vi "hold_data.vi"(7 "holda_data_mod":T2, 8 "Error In":errorcluster, 10 "config":T1={"rate"=1652.0, "duration"=1.0, "thr"=100.0, "preTrigger"=100.0, "cutoff"=-3.0, "Filtro"=enum."Desativado", "highPass"=1000.0, "lowPass"=1000.0, "updateTime"=50.0} {"updateTime" format="%#_g ms"; "lowPass" format="%#_g Hz"; "highPass" format="%#_g Hz"; "cutoff" format="%#_g dB"; "preTrigger" format="%#_g ms"; "thr" format="%#_g N"; "duration" format="%#_g s"; "rate" min=1652.0 max=51200.0 format="%#_g Hz"}, 11 "data":dbl[][](array[numeric])) -> (0 "Error Out":errorcluster, 3 "finished":bool)   [LabVIEW 2016]
uses:
  hold_data_mods.ctl
  MainFGV/Settings/Advanced/AdvancedConfig.ctl
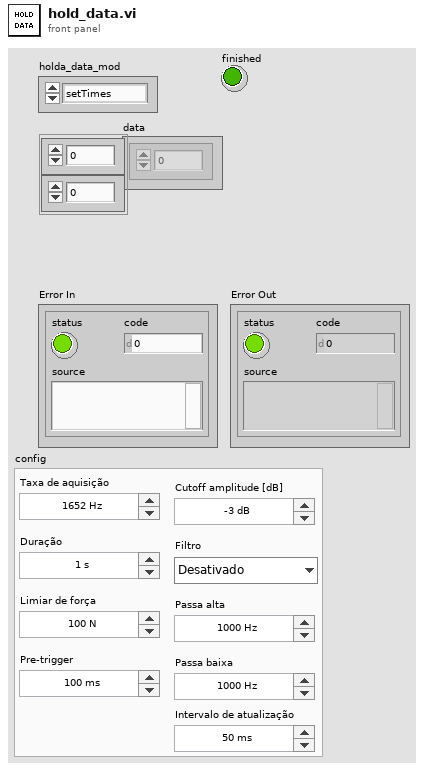
[diagram p1: front panel]
types:
  T1 = typedef "AdvancedConfig.ctl" = cluster{"rate":dbl, "duration":dbl, "thr":dbl, "preTrigger":dbl, "cutoff":dbl, "Filtro":enum16{"Desativado", "Passa banda", "Passa alta", "Passa baixa"}, "highPass":dbl, "lowPass":dbl, "updateTime":dbl}
  T2 = typedef "hold_data_mods.ctl" = enum16{"setTimes", "HoldPreTrigger", "HoldData"}
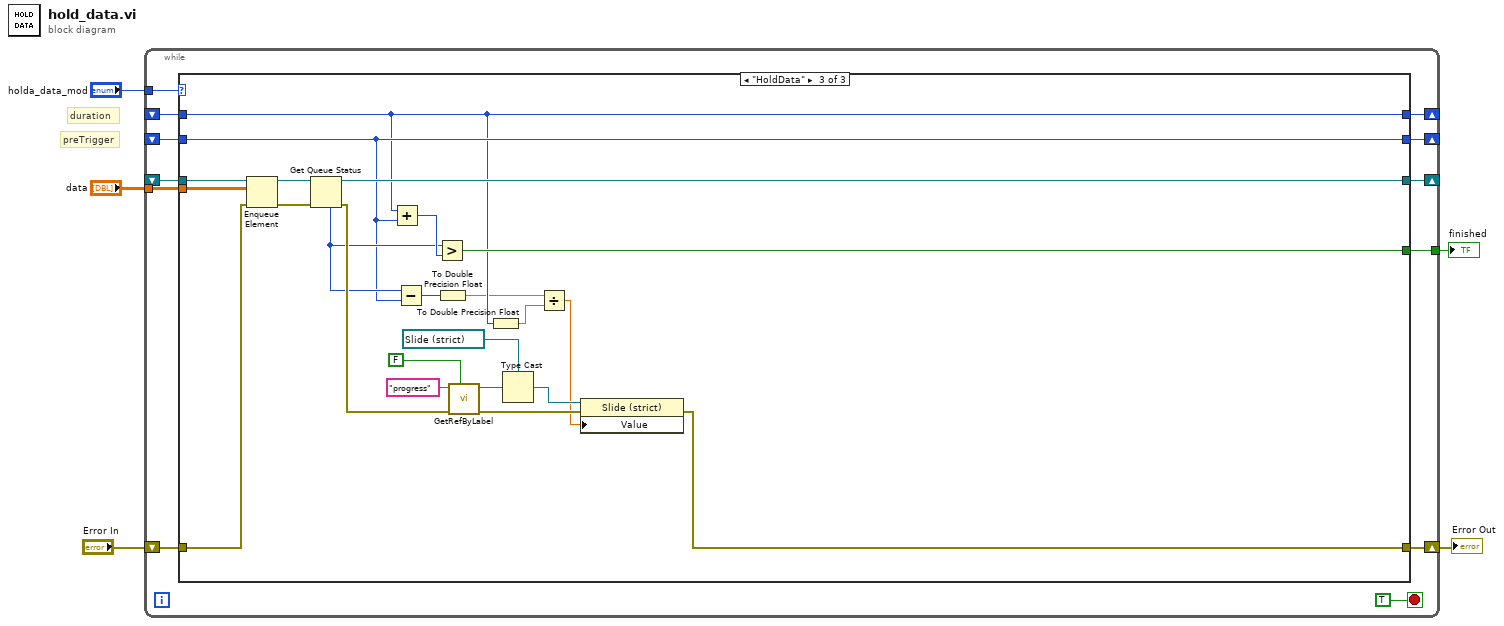
[diagram p0: block diagram]
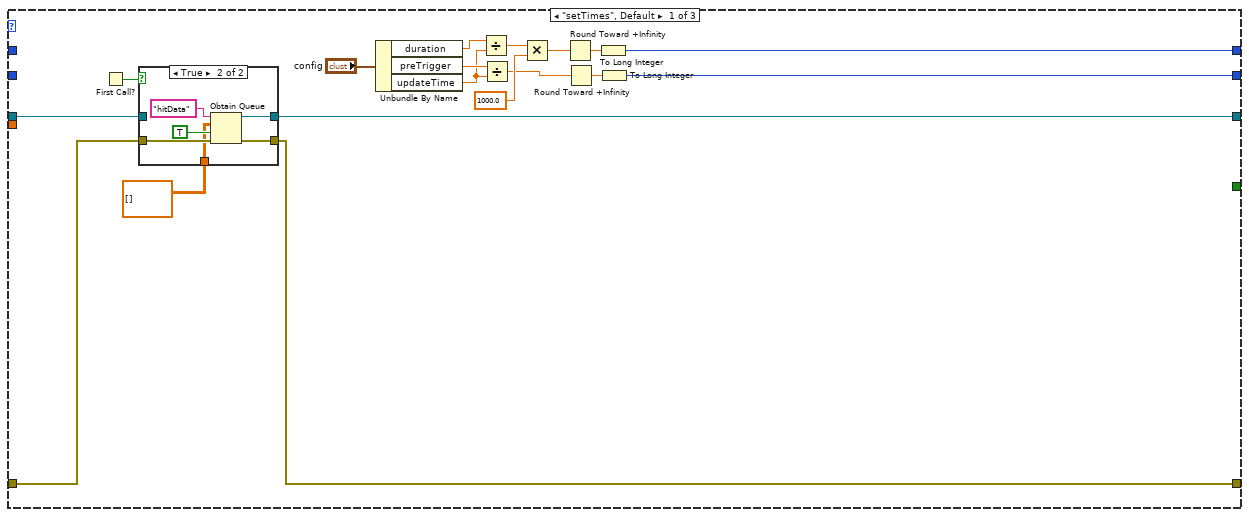
[diagram p2: hidden frame]
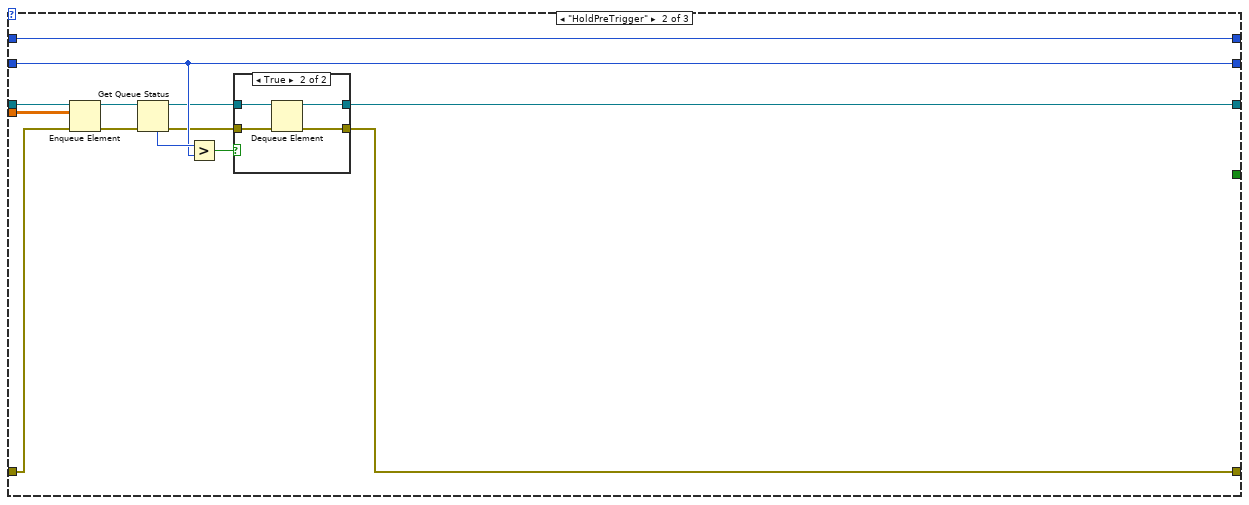
[diagram p4: hidden frame]
diagram:
  # "duration"
  # "preTrigger"
  n1 = while {
    tunnel: "holda_data_mod" -> [w16]
    shift-right: [w15] -> _
    shift-left: _ -> [w14]
    shift-right: [w12] -> w3
    shift-left: "Error In" -> [w13]
    shift-right: [w11] -> _
    shift-left: _ -> [w10]
    tunnel: "data" -> [w9]
    shift-right: [w8] -> _
    shift-left: _ -> [w7]
    tunnel: [w6] -> w1
    stop <- TRUE stop-if-true
    n2 = case shown="\"HoldData\"" w16 {
      tunnel: [w32 w55 w69] -> w15
      tunnel: w14 -> [_ w55 w69]
      tunnel: w13 -> [w31 w50 w83]
      tunnel: [w29 w46 w71] -> w12
      tunnel: [w30 w45 w80] -> w11
      tunnel: w10 -> [w27 w53 w85]
      tunnel: w9 -> [_ w49 w84]
      tunnel: [w22 w44 w67] -> w8
      tunnel: w7 -> [_ w44 w67]
      tunnel: [_ _ w78] -> w6
      frame "setTimes", Default {
        n3 = First Call?() -> (First Call?: T/F=w28:bool)
        n4 = case shown="True" w28 {
          tunnel: w31 -> [w37 w43]
          tunnel: [w36 w41] -> w30
          tunnel: [w37 w40] -> w29
          tunnel: w27 -> [w36 _]
          tunnel: dbl[][] [] ("data") -> [_ w38]
          frame False {
          }
          frame True {
            n5 = Obtain Queue(name (unnamed)="hitData", element data type=w38, create if not found? (T)=TRUE, error in (no error)=w43) -> (queue out=w41:refnum<queue>, error out=w40:errorcluster)  [unwired: 1 in, 1 out]
          }
        }
        n6 = Unbundle By Name("config") -> ("duration"=w24:dbl, "preTrigger"=w34:dbl, "updateTime"=w23:dbl)
        n7 = Divide(x=w24, y=w23) -> (x/y=w20:dbl)
        n8 = Divide(x=w34, y=w23) -> (x/y=w18:dbl)
        n9 = Multiply(x=w20, y=1000.0) -> (x*y=w21:dbl)
        n10 = Round Toward +Infinity(x=w21) -> (ceil(x): smallest int >= x=w25:dbl)
        n11 = Round Toward +Infinity(x=w18) -> (ceil(x): smallest int >= x=w33:dbl)
        n12 = To Long Integer(number=w25) -> (32bit integer=w22:i32)
        n13 = To Long Integer(number=w33) -> (32bit integer=w32:i32)
      }
      frame "HoldPreTrigger" {
        n14 = Enqueue Element(queue=w53, element=w49, error in (no error)=w50) -> (queue out=w52:refnum<queue>, error out=w51:errorcluster)  [unwired: 1 in, 1 out]
        n15 = Get Queue Status(queue=w52, error in (no error)=w51) -> (queue out=w47:refnum<queue>, error out=w48:errorcluster, # elements in queue=w56:i32)  [unwired: 1 in, 5 out]
        n16 = Greater?(x=w56, y=w55) -> (0:w54:bool)
        n17 = case shown="True" w54 {
          tunnel: w48 -> [w57 w62]
          tunnel: w47 -> [w58 w61]
          tunnel: [w57 w60] -> w46
          tunnel: [w58 w59] -> w45
          frame False {
          }
          frame True {
            n18 = Dequeue Element(queue=w61, error in (no error)=w62) -> (queue out=w59:refnum<queue>, error out=w60:errorcluster)  [unwired: 1 in, 2 out]
          }
        }
      }
      frame "HoldData" {
        n19 = Enqueue Element(queue=w85, element=w84, error in (no error)=w83) -> (queue out=w82:refnum<queue>, error out=w81:errorcluster)  [unwired: 1 in, 1 out]
        n20 = Get Queue Status(queue=w82, error in (no error)=w81) -> (queue out=w80:refnum<queue>, error out=w77:errorcluster, # elements in queue=w70:i32)  [unwired: 1 in, 5 out]
        n21 = Add(x=w67, y=w69) -> (x+y=w79:i32)
        n22 = Subtract(x=w70, y=w69) -> (x-y=w68:i32)
        n23 = Greater?(x=w70, y=w79) -> (0:w78:bool)
        n24 = To Double Precision Float(number=w68) -> (double precision float=w65:dbl)
        n25 = call "GetRefByLabel.vi"("InsideTab"=FALSE, "error in"=w77, "Label"="progress") -> ("error out"=w74:errorcluster, "Ctl Refnum"=w75:refnum<vi>)  [unwired: 6 in, 1 out]
        n26 = To Double Precision Float(number=w67) -> (double precision float=w66:dbl)
        n27 = Type Cast(type=refnum<vi> refnum ("progress"), x=w75) -> (*(type *) &x=w72:refnum<vi>)
        n28 = Divide(x=w65, y=w66) -> (x/y=w64:dbl)
        n29 = property class="Slide (strict)"(reference=w72, error in=w74, "Value"=w64) -> (error out=w71:errorcluster)  [unwired: 1 out]
      }
    }
  }
  "Error Out" <- w3
  "finished" <- w1
